vi "Average Data.vi"(8 "error in":errorcluster, 11 "Scan Driver.lvclass":refnum<class "Scan Driver.lvclass">) -> (0 "error out":errorcluster, 3 "Scan Driver.lvclass 2":refnum<class "Scan Driver.lvclass">)   [LabVIEW 2015, in "Scan Driver.lvclass"]
uses:
  Scan Driver.lvclass
  Scan Driver.lvclass/Scan Driver.ctl
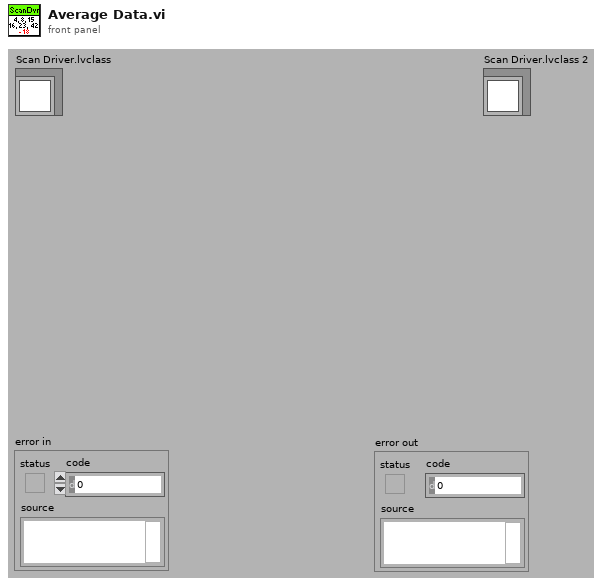
[diagram p1: front panel]
types:
  T1 = typedef "Readable.lvclass/Data Store.ctl" = T2[][]
  T2 = typedef "Readable.lvclass/Data Point.ctl" = cluster{"t":T3, "x":T4}
  T3 = typedef "Readable.lvclass/Time.ctl" = timestamp
  T4 = typedef "Readable.lvclass/X.ctl" = dbl
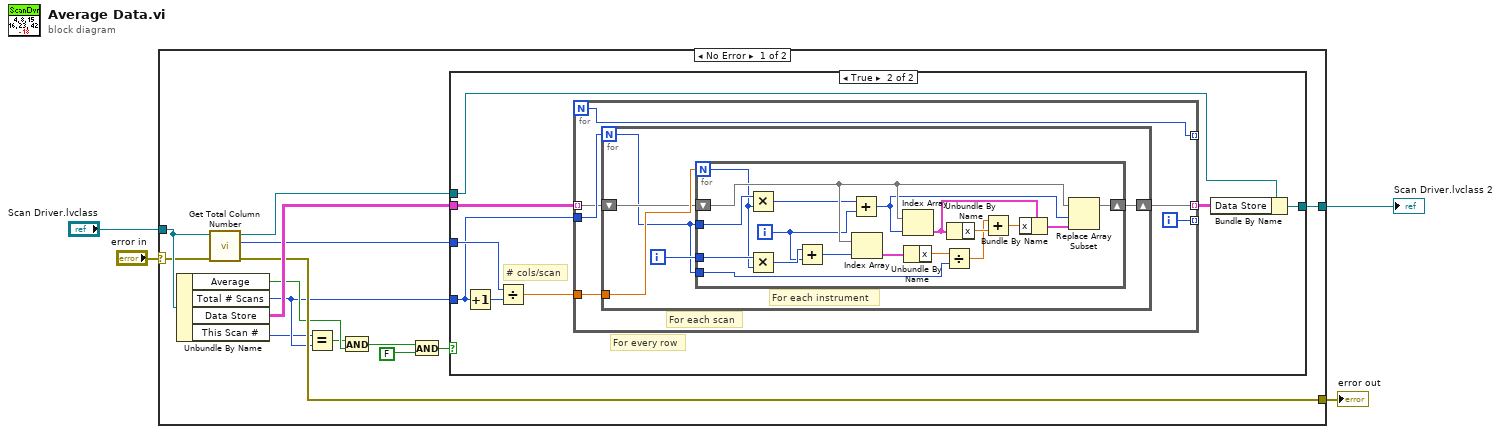
[diagram p0: block diagram]
diagram:
  n1 = case shown="No Error" "error in" {
    selector: "error in" -> [w15 w57]
    tunnel: [w14 w57] -> w3
    tunnel: [w12 w58] -> w2
    tunnel: "Scan Driver.lvclass" -> [w17 w58]
    frame No Error {
      n2 = Unbundle By Name(w17) -> ("Average"=w10:bool, "Total # Scans"=w9:u32, "Data Store"=w18:T1, "This Scan #"=w8:u32)
      n3 = call "Get Total Column Number.vi"("error in (no error)"=w15, "Scan Driver.lvclass"=w17) -> ("error out"=w14:errorcluster, "# of Columns"=w16:i32, "Scan Driver.lvclass"=w13:refnum<class "Scan Driver.lvclass">)  [unwired: 7 in]
      n4 = Equal?(x=w8, y=w9) -> (x = y?=w7:bool)
      n5 = And(x=w7, y=w10) -> (x .and. y?=w11:bool)
      n6 = And(x=w11, y=FALSE) -> (x .and. y?=w6:bool)
      n7 = case shown="True" w6 {
        tunnel: w9 -> [_ w24]
        tunnel: w18 -> [_ w27]
        tunnel: w16 -> [_ w26]
        tunnel: w13 -> [w19 w22]
        tunnel: [w19 w21] -> w12
        frame False {
        }
        frame True {
          # "For every row"
          # "# cols/scan"
          n8 = Increment(x=w24) -> (x+1=w25:u32)
          n9 = Divide(x=w26, y=w25) -> (x/y=w23:dbl)
          n10 = for {
            N -> [w28]
            tunnel: w27 -> [w31] mode=indexing
            tunnel: w24 -> [w33]
            tunnel: w23 -> [w32]
            tunnel: [w30] -> w20 mode=indexing
            tunnel: [w29] -> _ mode=indexing
            tunnel: [w28] -> _ mode=indexing
            i -> [w29]
            # "For each scan"
            n11 = for {
              N: w33 -> [w34]
              tunnel: w32 -> [w38]
              shift-right: [w35] -> w30
              shift-left: w31 -> [w37]
              i -> [w36]
              # "For each instrument"
              n12 = for {
                N: w38 -> [w51]
                tunnel: w36 -> [w56]
                tunnel: w34 -> [w52]
                shift-right: [w43] -> w35
                shift-left: w37 -> [w54]
                tunnel: w34 -> [w39]
                i -> [w49]
                n13 = Multiply(x=w52, y=w51) -> (x*y=w50:i32)
                n14 = Multiply(x=w56, y=w51) -> (x*y=w55:i32)
                n15 = Add(x=w55, y=w49) -> (x+y=w53:i32)
                n16 = Add(x=w50, y=w49) -> (x+y=w44:i32)
                n17 = Index Array(array=w54, index=w53) -> (element=w48:T2)
                n18 = Index Array(array=w54, index=w44) -> (element=w46:T2)
                n19 = Unbundle By Name(w48) -> ("x"=w40:T4)
                n20 = Divide(x=w40, y=w39) -> (x/y=w41:T4)
                n21 = Unbundle By Name(w46) -> ("x"=w42:T4)
                n22 = Add(x=w41, y=w42) -> (x+y=w47:T4)
                n23 = Bundle By Name(cluster=w46, "x"=w47) -> (w45:T2)
                n24 = Replace Array Subset(array=w54, new element=w45, index=w44) -> (w43:T2[])
              }
            }
          }
          n25 = Bundle By Name(cluster=w22, "Data Store"=w20) -> (w21:refnum<class "Scan Driver.lvclass">)
        }
      }
    }
    frame Error {
    }
  }
  "Scan Driver.lvclass 2" <- w2
  "error out" <- w3
